vi "Test Process Helper Loop Stopped when Process Stopped.vi"(8 "error in (no error)":errorcluster, 11 "Helper Loop Test In":refnum<class "Process Test.lvclass">) -> (0 "error out":errorcluster, 3 "Helper Loop Test Out":refnum<class "Process Test.lvclass">)   [LabVIEW 2020, in "Process Test.lvclass"]
uses:
  Process Test.lvclass
  C:/Program Files (x86)/National Instruments/LabVIEW 2020/vi.lib/Astemes/LUnit/Test Case.lvclass
  Framework/Helper Loop/Helper Loop.lvclass
  Framework/Process/Process.lvclass/Process.ctl
  <vilib>/Astemes/LUnit/Test Case.lvclass/Test Case.ctl
  <vilib>/Astemes/LUnit/LUnit Assertion Result.lvclass/LUnit Assertion Result.ctl
  <vilib>/Astemes/LUnit/LUnit Test Case Result.lvclass/LUnit Test Case Result.ctl
  <vilib>/Astemes/LUnit/LUnit Method Result.lvclass/LUnit Method Result.ctl
  4331ba45-8b7f-4b93-ba6e-ee1d1159701a.vi
  0f3fef22-4207-48e1-9b8b-17390fd24f63.vi
  e1ea3113-d8f4-4be9-9a25-bccd302f8800.vi
  Framework/Process/Public/Lifecycle/Get Lifecycle State.vi
  Framework/Broadcast Event Helpers/Dequeue Broadcast Message by Message Cluster.vi
  <vilib>/Astemes/LUnit/Palette/Pass.vi
  <vilib>/Astemes/LUnit/Palette/Fail.vi
  <vilib>/Astemes/LUnit/Compare Variants.vi
  <vilib>/Astemes/LUnit/Describe Comparison.vi
  <vilib>/Astemes/LUnit/Set Assertion Type.vi
  Framework/Process/Private/SubVIs/Wait for finish.vi
  Framework/Process/Protected/Messaging/Enqueue Message.vi
  Framework/Process/Private/SubVIs/Set Lifecycle State.vi
  <vilib>/Astemes/LUnit/Add test result.vi
  <vilib>/Astemes/LUnit/LUnit Write Message.vi
  <vilib>/Astemes/LUnit/LUnit Write Description.vi
  <vilib>/Astemes/LUnit/LUnit Write Skipped.vi
  <vilib>/Utility/error.llb/Clear Errors.vi
  Framework/Broadcast Event Helpers/Execution timer.vi
  <vilib>/Astemes/LUnit/LUnit Write Passed.vi
  <vilib>/Astemes/LUnit/Variant to string.vi
  <vilib>/Astemes/LUnit/LUnit Write Assertion Type.vi
  Framework/Process/Private/SubVIs/Handle Debug Data.vi
  <vilib>/Astemes/LUnit/LUnit Record Assertion Result.vi
  Framework/Logging/Log Debug.vi
  <vilib>/AdvancedString/1D String Array to Delimited String.vi
  <vilib>/Utility/High Resolution Relative Seconds.vi
  <vilib>/Astemes/LUnit/LUnit Aggregate Assertion Results.vi
  <vilib>/Astemes/LUnit/Assertion Result/LUnit Read Status.vi
  <vilib>/Astemes/LUnit/LUnit Read Message.vi
  <vilib>/Astemes/LUnit/LUnit Read Description.vi
  <vilib>/Astemes/LUnit/Method Result/LUnit Merge Status.vi
  <vilib>/Astemes/LUnit/LUnit Concatenate result strings.vi
  <vilib>/Utility/error.llb/Error Cluster From Error Code.vi
  Framework/Broadcast Event Helpers/Dequeue Broadcast Message.vi
  <vilib>/Utility/Data Type/Get Type Information.vi
  <vilib>/Utility/LVClass/Get LV Class Name.vi
  Framework/Process/Public/Read Name.vi
  <vilib>/Astemes/LUnit/LUnit Assertion Result.lvclass
  Framework/Process/Process.lvclass
  Process Test.lvclass/Process Test.ctl
  <vilib>/Astemes/LUnit/Test Case.lvclass
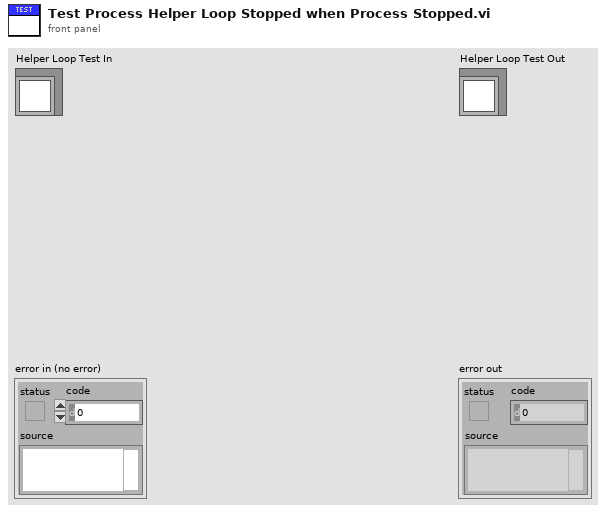
[diagram p1: front panel]
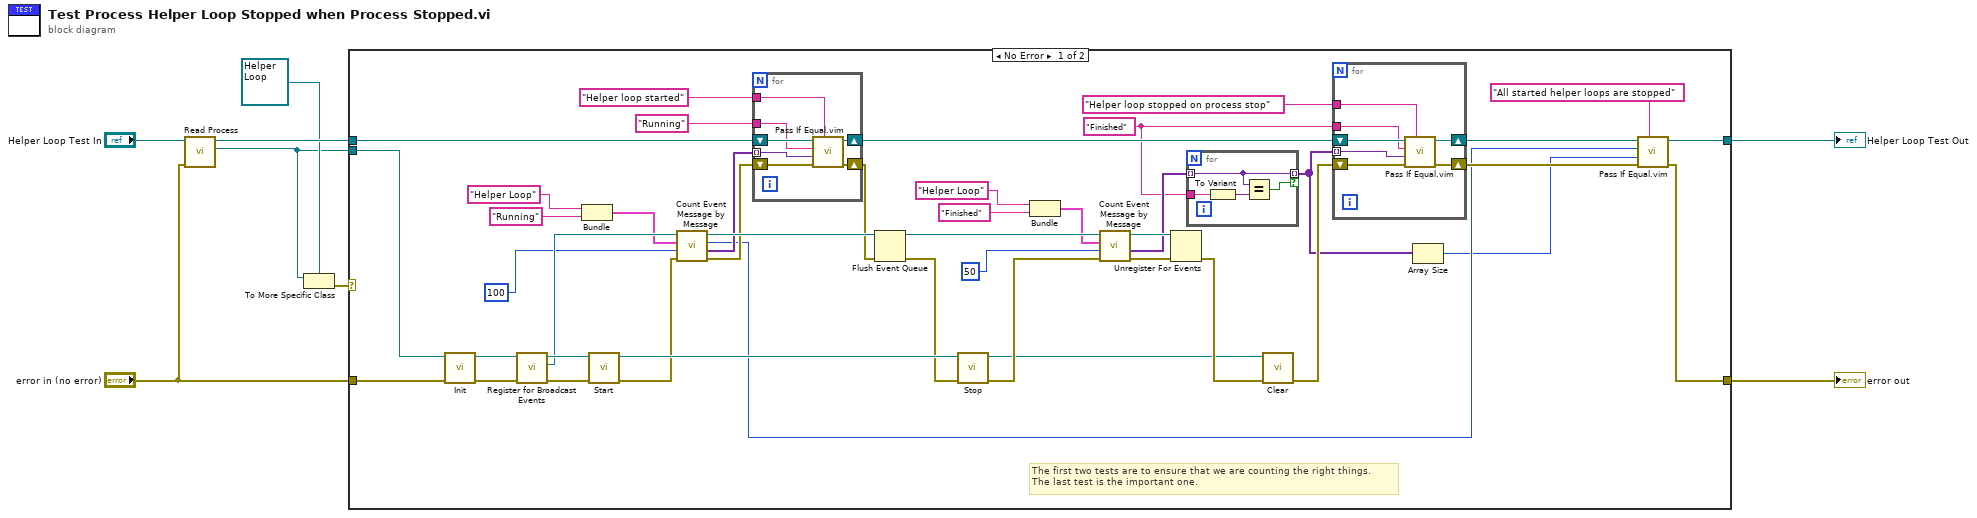
[diagram p0: block diagram]
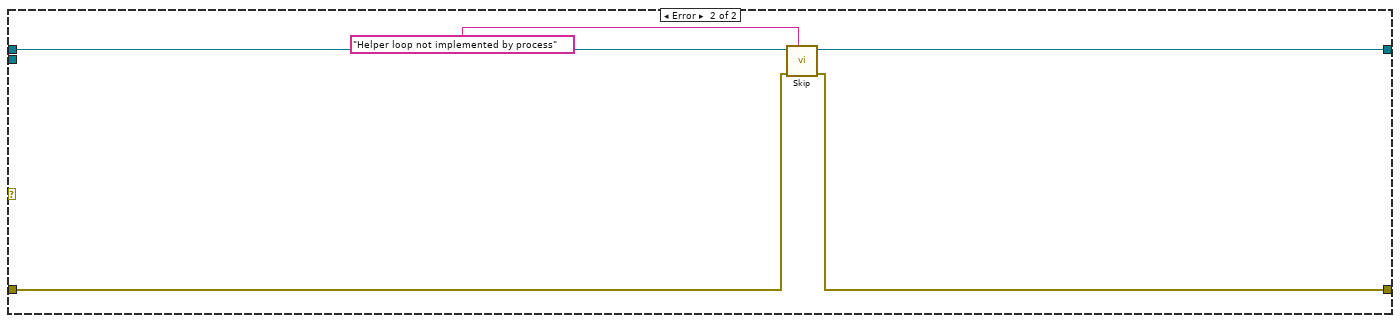
[diagram p2: hidden frame]
diagram:
  n1 = call "Read Process.vi"("error in (no error)"="error in (no error)", "Process Test in"="Helper Loop Test In") -> ("Process.lvclass"=w1:refnum<class "Process.lvclass">, "Process Test out"=w5:refnum<class "Process Test.lvclass">)  [unwired: 7 in, 1 out]
  n2 = To More Specific Class(target class=refnum<class "Helper Loop.lvclass"> refnum ("Helper Loop.lvclass"), reference=w1) -> (error out=w3:errorcluster)  [unwired: 1 in, 1 out]
  n3 = case shown="No Error" w3 {
    tunnel: [w23 w74] -> w8
    tunnel: "error in (no error)" -> [w46 w73]
    tunnel: [w21 w72] -> w7
    tunnel: w5 -> [w32 w75]
    tunnel: w1 -> [w38 _]
    frame No Error {
      w17 = "Finished" ("Description")
      # "The first two tests are to ensure that we are counting the right things. \nThe last test is the important one."
      n4 = call-dynamic "Init.vi"("error in (no error)"=w46, "Process In"=w38) -> ("error out"=w51:errorcluster, "Process Out"=w52:refnum<class "Process.lvclass">)  [unwired: 8 in]
      n5 = call "Register for Broadcast Events.vi"("error in (no error)"=w51, "Process In"=w52) -> ("error out"=w49:errorcluster, "Event Registration Refnum Out"=w37:refnum<event-registration>, "Process Out"=w50:refnum<class "Process.lvclass">)  [unwired: 7 in]
      n6 = Bundle("y"="Helper Loop", "Description"="Running") -> (w14:cluster{"y":string, "Description":string})  [unwired: 1 in]
      n7 = call "Start.vi"("error in (no error)"=w49, "Process In"=w50) -> ("error out"=w35:errorcluster, "Process Out"=w48:refnum<class "Process.lvclass">)  [unwired: 7 in, 1 out]
      n8 = call "Count Event Message by Message.vi"("error in (no error)"=w35, "Timeout"=100 ("Timeout (-1)"), "Message"=w14, "Event Registration Refnum in"=w37) -> ("error out"=w30:errorcluster, "Message Data"=w26:variant[], "Count"=w20:i32, "Event Registration Refnum out"=w36:refnum<event-registration>)  [unwired: 4 in]
      n9 = for {
        tunnel: "Helper loop started" ("Description") -> [w59]
        tunnel: "Running" ("Description") -> [w58]
        shift-right: [w63] -> w33
        shift-left: w32 -> [w62]
        shift-right: [w60] -> w29
        shift-left: w30 -> [w61]
        tunnel: w26 -> [w57] mode=indexing
        n10 = call "Pass If Equal.vim"("Description"=w59, "error in (no error)"=w61, "Actual"=w57, "Expected"=w58, "LUnit Test Case In"=w62) -> ("error out"=w60:errorcluster, "LUnit Test Case Out"=w63:refnum<class "Process Test.lvclass">)  [unwired: 5 in]
      }
      n11 = Flush Event Queue(0:w36, 3:w29) -> (8:w43:refnum<event-registration>, 11:w42:errorcluster)  [unwired: 4 in, 1 out]
      n12 = call "Stop.vi"("error in (no error)"=w42, "Process In"=w48) -> ("error out"=w41:errorcluster, "Process Out"=w40:refnum<class "Process.lvclass">)  [unwired: 7 in, 1 out]
      n13 = Bundle("y"="Helper Loop", "Description"="Finished") -> (w10:cluster{"y":string, "Description":string})  [unwired: 1 in]
      n14 = call "Count Event Message by Message.vi"("error in (no error)"=w41, "Timeout"=50 ("Timeout (-1)"), "Message"=w10, "Event Registration Refnum in"=w43) -> ("error out"=w39:errorcluster, "Message Data"=w18:variant[], "Event Registration Refnum out"=w45:refnum<event-registration>)  [unwired: 4 in, 1 out]
      n15 = Unregister For Events(event registration refnum=w45, error in=w39) -> (error out=w44:errorcluster)
      n16 = for {
        tunnel: [w53] -> w16 mode=indexing if=w55
        tunnel: w17 -> [w54]
        tunnel: w18 -> [w53] mode=indexing
        n17 = To Variant(anything=w54) -> (Variant=w56:variant)
        n18 = Equal?(x=w53, y=w56) -> (x = y?=w55:bool)
      }
      n19 = call-dynamic "Clear.vi"("error in (no error)"=w44, "Process In"=w40) -> ("error out"=w47:errorcluster)  [unwired: 9 in]
      n20 = for {
        tunnel: w16 -> [w67] mode=indexing
        shift-right: [w68] -> w22
        shift-left: w47 -> [w70]
        shift-right: [w69] -> w24
        shift-left: w33 -> [w66]
        tunnel: "Helper loop stopped on process stop" ("Description") -> [w65]
        tunnel: w17 -> [w64]
        n21 = call "Pass If Equal.vim"("Description"=w65, "error in (no error)"=w70, "Actual"=w67, "Expected"=w64, "LUnit Test Case In"=w66) -> ("error out"=w68:errorcluster, "LUnit Test Case Out"=w69:refnum<class "Process Test.lvclass">)  [unwired: 5 in]
      }
      n22 = Array Size(array=w16) -> (size(s)=w15:i32)
      n23 = call "Pass If Equal.vim"("Description"="All started helper loops are stopped", "error in (no error)"=w22, "Actual"=w15, "Expected"=w20, "LUnit Test Case In"=w24) -> ("error out"=w21:errorcluster, "LUnit Test Case Out"=w23:refnum<class "Process Test.lvclass">)  [unwired: 5 in]
    }
    frame Error {
      n24 = call <vilib>:"Skip.vi"("Description"="Helper loop not implemented by process", "error in (no error)"=w73, "LUnit Test Case In"=w75) -> ("error out"=w72:errorcluster, "LUnit Test Case Out"=w74:refnum<class "Process Test.lvclass">)  [unwired: 7 in]
    }
  }
  "error out" <- w7
  "Helper Loop Test Out" <- w8
